vi "ReadWrite.Data.Buffer.vi"(8 "error in (no error)":errorcluster, 9 "Offset":i32, 10 "Values":dbl[](array[numeric]), 11 "Ref":T1) -> (0 "error out":errorcluster)   [LabVIEW 2027, in "Data Access Engine.lvlib" / "Data Access Engine.lvclass"]
uses:
  Data Access Engine.lvclass
  Types/ReadWrite.DVR.ctl
  Access Type Classes/ReadWrite/ReadWrite.lvclass
  Access Type Classes/ReadWrite/ReadWrite.lvclass/ReadWrite.ctl
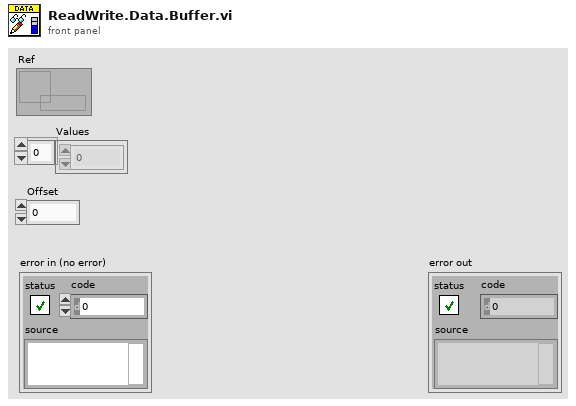
[diagram p1: front panel]
types:
  T1 = typedef "Data Access Engine.lvlib/Data Access Engine.lvclass/ReadWrite.DVR.ctl" = refnum<data-value>
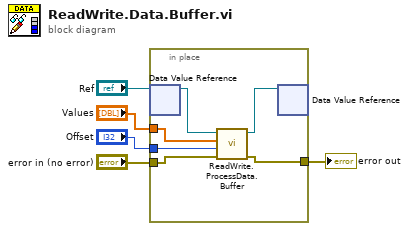
[diagram p0: block diagram]
diagram:
  n1 = in-place {
    in-place-border: "error in (no error)" -> [w8]
    in-place-border: "Values" -> [w7]
    in-place-border: "Offset" -> [w6]
    in-place-border: [w9] -> w1
    n2 = in-place-dvr #1("Ref") -> (w11:refnum<class "ReadWrite.lvclass">)  [unwired: 1 out]
    n3 = call "ReadWrite.ProcessData.Buffer.vi"("error in (no error)"=w8, "Offset"=w6, "Values"=w7, "ReadWrite in"=w11) -> ("error out"=w9:errorcluster, "ReadWrite out"=w10:refnum<class "ReadWrite.lvclass">)  [unwired: 6 in]
    n4 = in-place-dvr #1(w10) -> ()  [unwired: 2 out]
  }
  "error out" <- w1
